vi "Actor Core.vi"(8 "error in":errorcluster, 11 "Island Watch in":refnum<class "Island Watch.lvclass">) -> (0 "error out":errorcluster, 3 "Actor out":refnum<class "Actor.lvclass">)   [LabVIEW 2015, in "Island Watch Actor.lvlib" / "Island Watch.lvclass"]
doc: "(<B>Filename</B>: Actor Framework.lvlib:Actor.lvclass:Actor Core.vi)\n\nReceives messages to the actor, reacts to them, and initiates any error handling that may shut the actor down.\n\nDescendant classes may override this VI to append parallel tasks for the actor to complete while it handles messages. Overrides use the Call Parent Method node."
uses:
  Island Watch.lvclass
  <vilib>/ActorFramework/Actor/Actor.lvclass
  <vilib>/ActorFramework/Actor/Actor.lvclass/Actor.ctl
  <vilib>/ActorFramework/Message Enqueuer/Message Enqueuer.lvclass/Message Enqueuer.ctl
  Island Watch.lvclass/Island Watch.ctl
  <vilib>/ActorFramework/Message Enqueuer/Init from Existing Queue.vi
  <vilib>/ActorFramework/Message Enqueuer/Enqueue.vi
  <vilib>/ActorFramework/Message Priority Queue/Priority Enqueue.vi
  <vilib>/ActorFramework/Message Enqueuer/Message Enqueuer.lvclass
  Island Watch Messages/Read Check Msg/Read Check Msg.lvclass
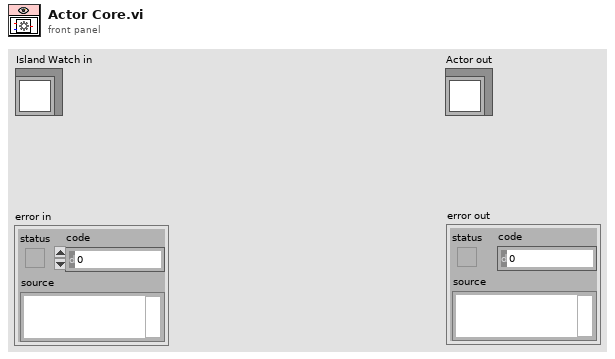
[diagram p1: front panel]
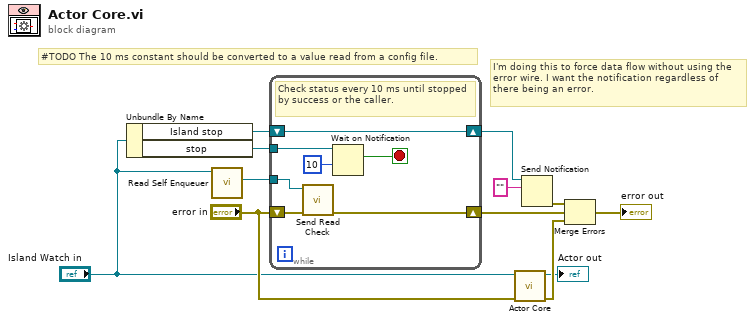
[diagram p0: block diagram]
diagram:
  # "#TODO The 10 ms constant should be converted to a value read from a config file."
  # "I'm doing this to force data flow without using the error wire. I want the notification regardless of there being an error."
  n1 = Unbundle By Name("Island Watch in") -> ("Island stop"=w4:refnum<notifier>, "stop"=w10:refnum<notifier>)
  n2 = call <vilib>:"Read Self Enqueuer.vi"("Actor"="Island Watch in") -> ("Self Enqueuer"=w5:refnum<class "Message Enqueuer.lvclass">)  [unwired: 10 in]
  n3 = while {
    tunnel: w10 -> [w19]
    shift-right: [w15] -> w8
    shift-left: "error in" -> [w16]
    tunnel: w5 -> [w14]
    shift-right: [w13] -> w2
    shift-left: w4 -> [w13]
    stop <- w17 stop-if-true
    # "Check status every 10 ms until stopped by success or the caller."
    n4 = call "Send Read Check.vi"("error in (no error)"=w16, "Message Enqueuer"=w14) -> ("error out"=w15:errorcluster)  [unwired: 8 in, 1 out]
    n5 = Wait on Notification(notifier=w19, timeout in ms (-1)=10) -> (notification=w17:bool)  [unwired: 2 in, 3 out]
  }
  n6 = call-parent "Actor Core.vi"("error in"="error in", "Actor in"="Island Watch in") -> ("error out"=w12:errorcluster, "Actor out"=→"Actor out":refnum<class "Actor.lvclass">)  [unwired: 8 in]
  n7 = Send Notification(notification="", notifier=w2) -> (error out=w1:errorcluster)  [unwired: 1 in, 1 out]
  n8 = Merge Errors(w1, w8, w12) -> (→"error out":errorcluster)
